vi "csm_lumikki_instron_stopLogging.vi"() -> ()   [LabVIEW 2009]
panel:
  out "stopLoggingOut":bool
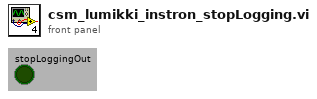
[diagram p1: front panel]
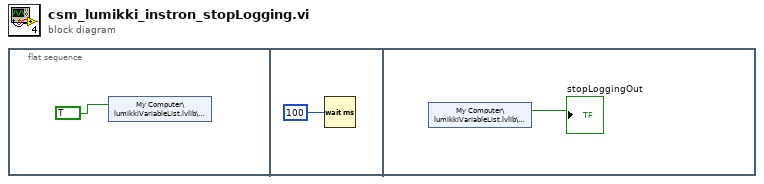
[diagram p0: block diagram]
diagram:
  n1 = flat-sequence {
    frame #0 {
      n2 = shared-variable "My Computer\\lumikkiVariableList.lvlib\\stopLogging"(TRUE ("Busy")) -> ()  [unwired: 1 in, 1 out]
    }
    frame #1 {
      n3 = Wait (ms)(milliseconds to wait=u32 100) -> ()  [unwired: 1 out]
    }
    frame #2 {
      n4 = shared-variable "My Computer\\lumikkiVariableList.lvlib\\stopLogging"() -> (→"stopLoggingOut":bool)  [unwired: 1 in, 1 out]
    }
  }
